vi "Pos_Modf.vi"() -> ()   [LabVIEW 2017]
panel:
  in  "Pos_Modf":T1
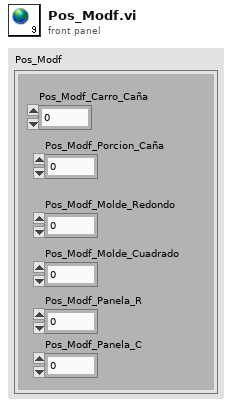
[diagram p1: front panel]
types:
  T1 = cluster{"Pos_Modf_Carro_Caña":i32, "Pos_Modf_Porcion_Caña":i32, "Pos_Modf_Molde_Redondo":i32, "Pos_Modf_Molde_Cuadrado":i32, "Pos_Modf_Panela_R":i32, "Pos_Modf_Panela_C":i32}
diagram:
